vi "Connect.vi"(8 "error in":errorcluster, 11 "DAQ970 in":refnum<class "DAQ970.lvclass">) -> (0 "error out":errorcluster, 3 "DAQ970 out":refnum<class "DAQ970.lvclass">)   [LabVIEW 2019, in "DAQ970.lvlib" / "DAQ970.lvclass"]
uses:
  Library/DAQ970.lvclass
  C:/Users/Public/Documents/Development/builds/Instruments/Instruments.lvlibp/Library/Instruments.lvclass
  Library/DAQ970.lvclass/DAQ970.ctl
  builds/Instruments/Instruments.lvlibp/Accessors/Read Resource.vi
  <instrlib>/Keysight DAQ970/Keysight DAQ970.lvlib
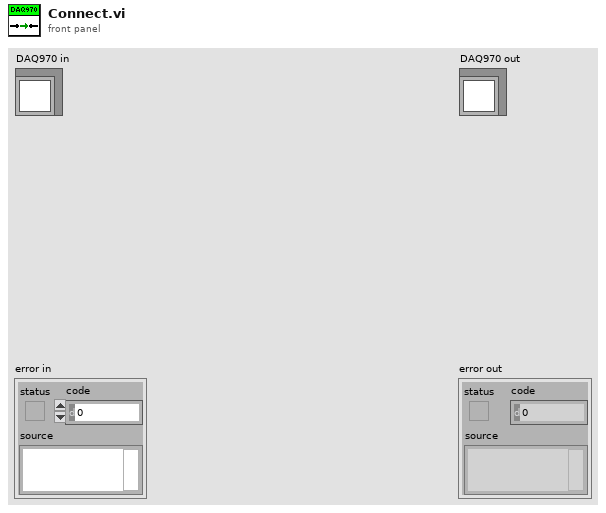
[diagram p1: front panel]
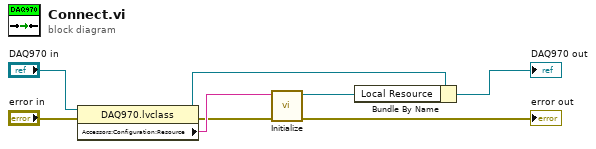
[diagram p0: block diagram]
diagram:
  n1 = property class="DAQ970.lvclass"(reference="DAQ970 in", error in="error in") -> (reference out=w3:refnum<class "DAQ970.lvclass">, error out=w1:errorcluster, "Accessors:Configuration:Resource"=w4:string)
  n2 = call <instrlib>:"Initialize.vi"("error in (no error)"=w1, "resource string"=w4) -> ("error out"=→"error out":errorcluster, "instrument handle out"=w2:refnum<k15>)  [unwired: 8 in]
  n3 = Bundle By Name(cluster=w3, "Local Resource"=w2) -> (→"DAQ970 out":refnum<class "DAQ970.lvclass">)
